vi "Get Ball Pose.vi"(11 "Detection Ball":T1) -> (3 "Pose":T2)   [LabVIEW 2017]
uses:
  <vilib>/Analysis/Matrix/NI_Matrix.lvlib
  <vilib>/Analysis/Matrix/Numeric/Conversions/Array To Matrix - RA.vi
  <vilib>/Analysis/Matrix/Datatypes/RealMatrix.ctl
  SSL Detection Ball w ID.ctl
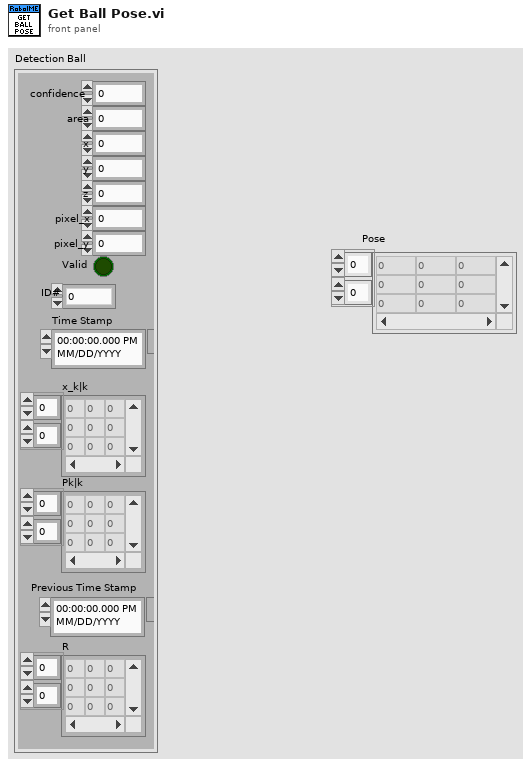
[diagram p1: front panel]
types:
  T1 = typedef "SSL Detection Ball w ID.ctl" = cluster{"x":sgl, "area":u32, "confidence":sgl, "y":sgl, "z":sgl, "pixel_x":sgl, "pixel_y":sgl, "Valid":bool, "Time Stamp":timestamp, "x_k|k":T2, "Pk|k":T2, "ID#":u32, "Previous Time Stamp":timestamp, "R":T2}
  T2 = typedef "NI_Matrix.lvlib/RealMatrix.ctl" = dbl[][]
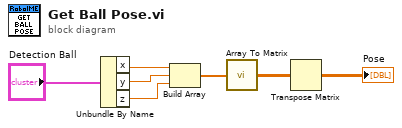
[diagram p0: block diagram]
diagram:
  n1 = Unbundle By Name("Detection Ball") -> ("x"=w5:sgl, "y"=w6:sgl, "z"=w7:sgl)
  n2 = Build Array(w5, w6, w7) -> (w4:sgl[])
  n3 = call-poly <vilib>:"Array To Matrix.vi"("Real 1D Array"=w4) -> ("Real Matrix (Column Vector)"=w3:T2)
  n4 = Transpose Matrix(1:w3) -> (0:→"Pose":T2)
